vi "GetMaxOrigDly.vi"(8 "错误输入（无错误）":errorcluster, 11 "当前通道序号":u8) -> (0 "错误输出":errorcluster, 3 "返回值":u32)   [LabVIEW 2014]
uses:
  X86Dll/ZXUTConfigMgr.dll
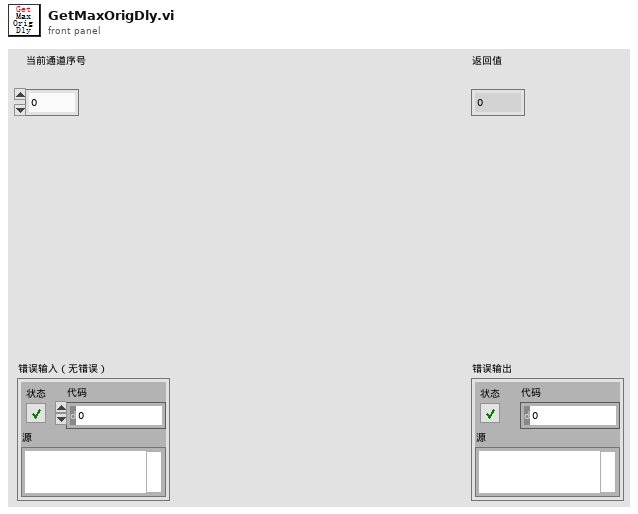
[diagram p1: front panel]
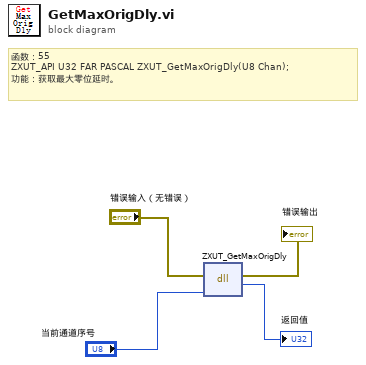
[diagram p0: block diagram]
diagram:
  # "函数：55\nZXUT_API U32\tFAR PASCAL ZXUT_GetMaxOrigDly(U8 Chan);\n功能：获取最大零位延时。"
  n1 = dll-call lib="D:/Software/Utrasonic on-line monitoring/X86Dll/ZXUTConfigMgr.dll" fn="ZXUT_GetMaxOrigDly"(error in="错误输入（无错误）", "Chan"="当前通道序号") -> (error out=→"错误输出":errorcluster, "返回值"=→"返回值":u32)  [unwired: 3 in, 1 out]
